vi "fix symbolic paths.vi"(11 "in":string) -> (3 "out":string)   [LabVIEW 2016]
uses:
  <vilib>/Utility/sysdir.llb/System Directory Type.ctl
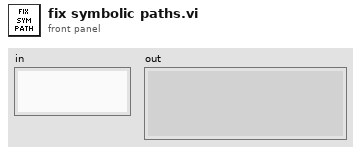
[diagram p1: front panel]
types:
  T1 = typedef "System Directory Type.ctl" = i32
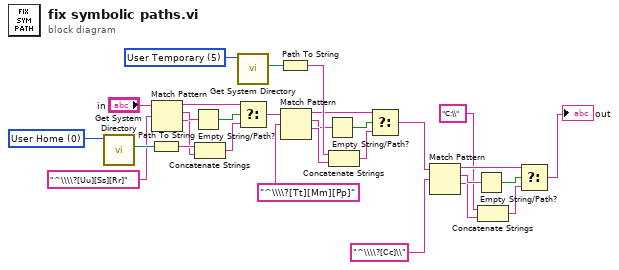
[diagram p0: block diagram]
diagram:
  w27 = T1 5 items=["User Home"=0, "User Desktop"=1, "User Documents"=2, "User Application Data"=3, "User Preferences"=4, "User Temporary"=5, "Public Documents"=6, "Public Application Data"=7, "Public Preferences"=8, "Public Cache"=13, "System Core Libraries"=9, "System Installed Libraries"=10, "Application Files"=11, "Boot Volume Root"=12] ("system directory type")
  w29 = T1 0 items=["User Home"=0, "User Desktop"=1, "User Documents"=2, "User Application Data"=3, "User Preferences"=4, "User Temporary"=5, "Public Documents"=6, "Public Application Data"=7, "Public Preferences"=8, "Public Cache"=13, "System Core Libraries"=9, "System Installed Libraries"=10, "Application Files"=11, "Boot Volume Root"=12] ("system directory type")
  n1 = call <vilib>:"Get System Directory.vi"("system directory type"=w29) -> ("system directory"=w28:path)  [unwired: 10 in]
  n2 = Path To String(path=w28) -> (string=w21:string)
  n3 = Match Pattern(string="in", regular expression="^\\\\?[Uu][Ss][Rr]" ("search string")) -> (before substring=w22:string, match substring=w24:string, after substring=w20:string)  [unwired: 1 in, 1 out]
  n4 = Empty String/Path?(string/path=w24) -> (empty?=w23:bool)
  n5 = Concatenate Strings(w21, w20) -> (w19:string)
  n6 = call <vilib>:"Get System Directory.vi"("system directory type"=w27) -> ("system directory"=w11:path)  [unwired: 10 in]
  n7 = Select(t=w22, s=w23, f=w19) -> (s? t:f=w12:string)
  n8 = Path To String(path=w11) -> (string=w16:string)
  n9 = Match Pattern(string=w12, regular expression="^\\\\?[Tt][Mm][Pp]" ("search string")) -> (before substring=w15:string, match substring=w13:string, after substring=w17:string)  [unwired: 1 in, 1 out]
  n10 = Empty String/Path?(string/path=w13) -> (empty?=w14:bool)
  n11 = Concatenate Strings(w16, w17) -> (w18:string)
  n12 = Select(t=w15, s=w14, f=w18) -> (s? t:f=w3:string)
  n13 = Match Pattern(string=w3, regular expression="^\\\\?[Cc]\\" ("search string")) -> (before substring=w6:string, match substring=w8:string, after substring=w5:string)  [unwired: 1 in, 1 out]
  n14 = Empty String/Path?(string/path=w8) -> (empty?=w7:bool)
  n15 = Concatenate Strings("C:\\" ("search string"), w5) -> (w4:string)
  n16 = Select(t=w6, s=w7, f=w4) -> (s? t:f=→"out":string)
